vi "sv_Check Data Valid (N Ch) [Octave Filtering].vi"(7 "reset filter (F)":bool, 8 "error in (no error)":errorcluster, 9 "midband frequency setting":T3, 10 "1/n octave settings":T2, 11 "scaled signal(s)":waveform(dbl)[](array[waveform])) -> (0 "error out":errorcluster, 2 "reset filter":bool, 3 "dup scaled signal(s)":waveform(dbl)[](array[waveform]))   [LabVIEW 2017, in "SoundVib_Octave_2014 standard.lvlib"]
uses:
  <vilib>/addons/Sound and Vibration/svt_Octave/SoundVib_Octave_2014 standard.lvlib
  <vilib>/addons/_NISVFA/_Shared subVIs/Controls/svc_Octave Standard.ctl
  <vilib>/addons/_NISVFA/_Shared subVIs/Common/svc_Check for Waveform Parameter Continuity (no state).vi
  <vilib>/addons/_NISVFA/_Shared subVIs/Common/svc_Get SV Channel Info.vi
  <vilib>/addons/_NISVFA/_Shared subVIs/Common/svc_Engineering Units to Unit Label.vi
  <vilib>/addons/_NISVFA/_Shared subVIs/Common/svc_Unit Label to Engineering Units.vi
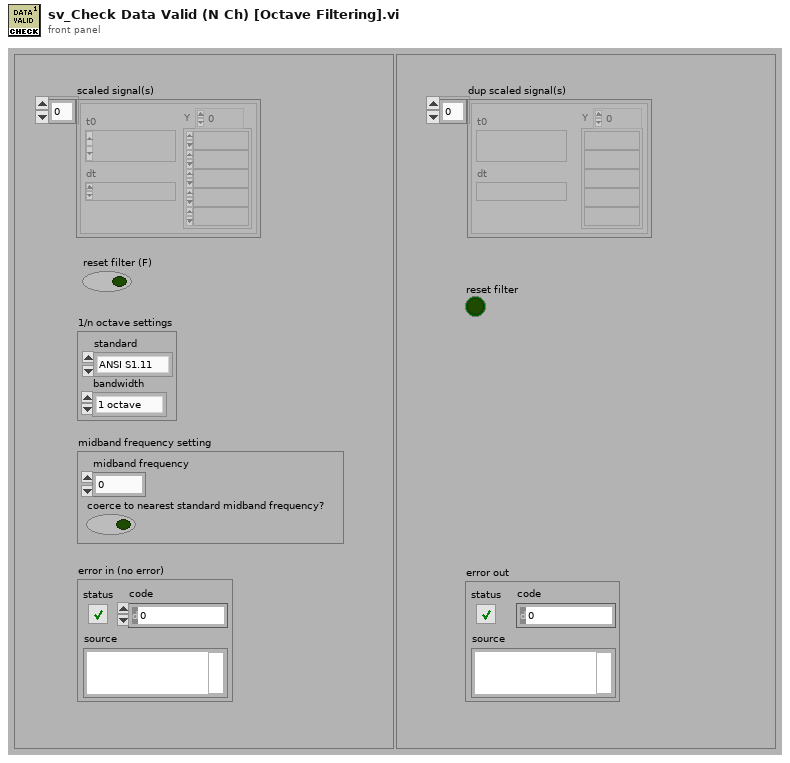
[diagram p1: front panel]
types:
  T1 = typedef "svc_Octave Standard.ctl" = enum16{"ANSI S1.11", "IEC 61260"}
  T2 = cluster{"standard":T1, "bandwidth":enum16{"1 octave", "1/3 octave", "1/6 octave", "1/12 octave", "1/24 octave"}}
  T3 = cluster{"midband frequency":dbl, "coerce to nearest standard midband frequency?":bool}
  T4 = cluster{"dt equal":bool, "array length equal":bool, "number channels change":bool}
  T5 = cluster{"dt":bool, "t0 continuity":bool, "array length":bool, "channel info":bool, "name":bool}
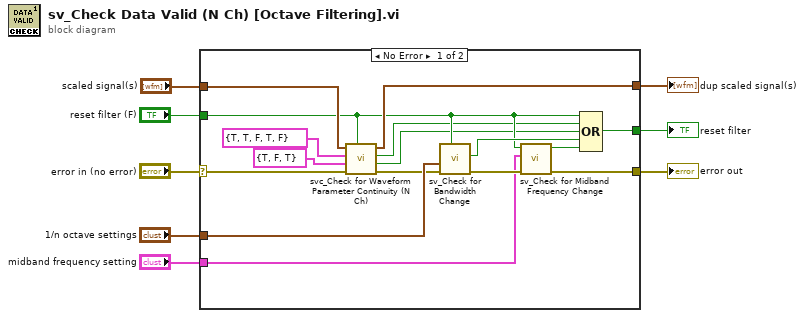
[diagram p0: block diagram]
diagram:
  n1 = case shown="No Error" "error in (no error)" {
    selector: "error in (no error)" -> [w17 w26]
    tunnel: "reset filter (F)" -> [w11 w27]
    tunnel: "midband frequency setting" -> [w23 _]
    tunnel: "1/n octave settings" -> [w21 _]
    tunnel: [w19 w26] -> w4
    tunnel: [w18 w27] -> w3
    tunnel: "scaled signal(s)" -> [w15 w25]
    tunnel: [w14 w25] -> w1
    frame No Error {
      n2 = call <vilib>:"svc_Check for Waveform Parameter Continuity (N Ch).vi"("restart averaging (F)"=w11, "error in (no error)"=w17, "checks for multichannel parameters"=T4 {"dt equal"=TRUE, "array length equal"=FALSE, "number channels change"=TRUE}, "checks for channel parameter change"=T5 {"dt"=TRUE, "t0 continuity"=TRUE, "array length"=FALSE, "channel info"=TRUE, "name"=FALSE}, "scaled signal(s)"=w15) -> ("error out"=w16:errorcluster, "multichannel parameter changed"=w10:bool, "waveform parameter changed"=w9:bool, "dup scaled signal(s)"=w14:waveform(dbl)[])  [unwired: 3 out]
      n3 = call <vilib>:"sv_Check for Bandwidth Change.vi"("reset filter (F)"=w11, "error in (no error)"=w16, "1/n octave settings"=w21) -> ("error out"=w24:errorcluster, "parameter has changed"=w20:bool)  [unwired: 6 in, 1 out]
      n4 = call <vilib>:"sv_Check for Midband Frequency Change.vi"("error in (no error)"=w24, "midband frequency setting"=w23, "reset filter (F)"=w11) -> ("error out"=w19:errorcluster, "parameter has changed"=w22:bool)  [unwired: 7 in]
      n5 = Compound Arithmetic op=OR(w11, w9, w10, w20, w22) -> (w18:bool)
    }
    frame Error {
    }
  }
  "error out" <- w4
  "reset filter" <- w3
  "dup scaled signal(s)" <- w1
